vi "Create.vi"(8 "error in (no error)":errorcluster, 11 "Serial in":refnum<class "Modbus Serial.lvclass">) -> (0 "error out":errorcluster, 3 "Serial out":refnum<class "Modbus Serial.lvclass">)   [LabVIEW 2021, in "Modbus Serial.lvclass"]
uses:
  Modbus Serial.lvclass
  Serial.lvclass
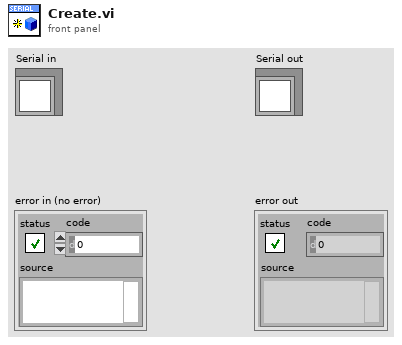
[diagram p1: front panel]
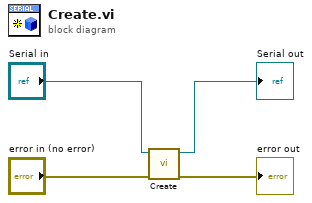
[diagram p0: block diagram]
diagram:
  n1 = call-parent "Create.vi"("error in (no error)"="error in (no error)", "Serial in"="Serial in") -> ("error out"=→"error out":errorcluster, "Serial out"=→"Serial out":refnum<class "Modbus Serial.lvclass">)  [unwired: 8 in]
